vi "Begin.vi"(8 "error in (no error)":errorcluster, 11 "Comp Pressure in":refnum<class "Comp Pressure.lvclass">) -> (0 "error out":errorcluster, 3 "Comp Pressure out":refnum<class "Comp Pressure.lvclass">)   [LabVIEW 2014, in "Comp Pressure.lvlib" / "Comp Pressure.lvclass"]
uses:
  Comp Pressure.lvclass
  Comp Pressure.lvclass/Comp Pressure.ctl
  Robot/Pressure/Pressure Class/Pressure.lvclass
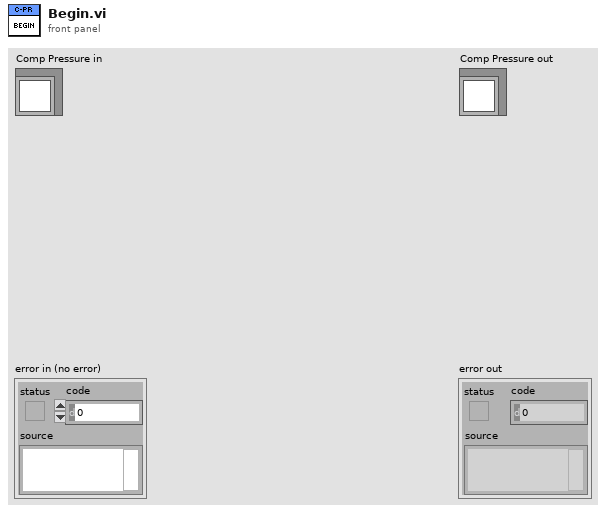
[diagram p1: front panel]
types:
  T1 = typedef "WPI_CompressorDevRef.ctl" = cluster{"DevStatus":errorcluster, "Pneumatics Control Module":u8}
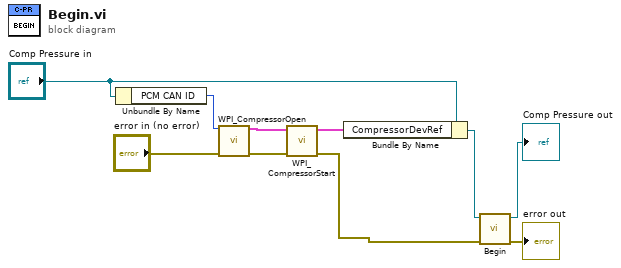
[diagram p0: block diagram]
diagram:
  n1 = Unbundle By Name("Comp Pressure in") -> ("PCM CAN ID"=w2:u8)
  n2 = call <vilib>:"WPI_CompressorOpen.vi"("Pneumatics Control Module (0)"=w2, "error in (no error)"="error in (no error)") -> ("CompressorDevRef"=w7:T1, "error out"=w8:errorcluster)  [unwired: 12 in]
  n3 = call <vilib>:"WPI_CompressorStart.vi"("error in (no error)"=w8, "CompressorDevRef"=w7) -> ("error out"=w1:errorcluster, "CompressorDevRef"=w4:T1)  [unwired: 8 in]
  n4 = Bundle By Name(cluster="Comp Pressure in", "CompressorDevRef"=w4) -> (w5:refnum<class "Comp Pressure.lvclass">)
  n5 = call-parent "Begin.vi"("error in (no error)"=w1, "Pressure in"=w5) -> ("error out"=→"error out":errorcluster, "Pressure out"=→"Comp Pressure out":refnum<class "Comp Pressure.lvclass">)  [unwired: 8 in]
